vi "In.vi"   [LabVIEW 2013]
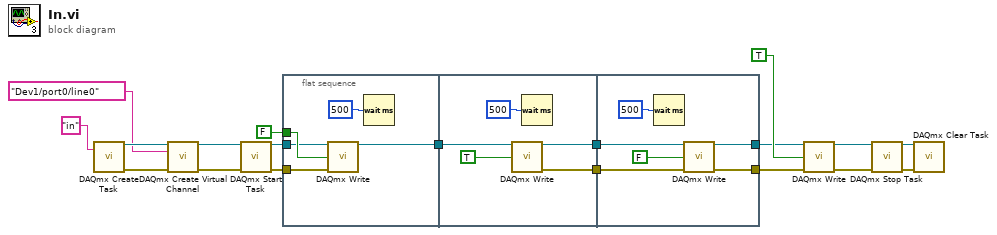
[diagram p0: block diagram]
diagram:
  n1 = call <vilib>:"DAQmx Create Task.vi"("new task name"="in") -> ("task out"=w15:refnum<k21>, "error out"=w13:errorcluster)  [unwired: 13 in]
  n2 = call-poly <vilib>:"DAQmx Create Virtual Channel.vi"("task in"=w15, "lines"=tag "Dev1/port0/line0", "error in"=w13) -> ("task out"=w12:refnum<k21>, "error out"=w11:errorcluster)  [unwired: 11 in]
  n3 = call <vilib>:"DAQmx Start Task.vi"("task/channels in"=w12, "error in"=w11) -> ("task out"=w10:refnum<k21>, "error out"=w7:errorcluster)  [unwired: 12 in]
  n4 = flat-sequence {
    tunnel: w10 -> [w20]
    tunnel: [w23] -> w19
    tunnel: w7 -> [w22]
    tunnel: FALSE ("data") -> [w21]
    tunnel: w19 -> [w28]
    tunnel: [w27] -> w18
    tunnel: [w25] -> w17
    tunnel: w18 -> [w34]
    tunnel: [w33] -> w8
    tunnel: w17 -> [w31]
    tunnel: [w30] -> w6
    frame #0 {
      n5 = call-poly <vilib>:"DAQmx Write.vi"("task/channels in"=w20, "data"=w21, "error in"=w22) -> ("task out"=w23:refnum<k21>)  [unwired: 10 in, 2 out]
      n6 = Wait (ms)(milliseconds to wait=u32 500) -> ()  [unwired: 1 out]
    }
    frame #1 {
      n7 = call-poly <vilib>:"DAQmx Write.vi"("task/channels in"=w28, "data"=TRUE) -> ("task out"=w27:refnum<k21>, "error out"=w25:errorcluster)  [unwired: 11 in, 1 out]
      n8 = Wait (ms)(milliseconds to wait=u32 500) -> ()  [unwired: 1 out]
    }
    frame #2 {
      n9 = Wait (ms)(milliseconds to wait=u32 500) -> ()  [unwired: 1 out]
      n10 = call-poly <vilib>:"DAQmx Write.vi"("task/channels in"=w34, "data"=FALSE, "error in"=w31) -> ("task out"=w33:refnum<k21>, "error out"=w30:errorcluster)  [unwired: 10 in, 1 out]
    }
  }
  n11 = call-poly <vilib>:"DAQmx Write.vi"("task/channels in"=w8, "data"=TRUE, "error in"=w6) -> ("task out"=w5:refnum<k21>, "error out"=w2:errorcluster)  [unwired: 10 in, 1 out]
  n12 = call <vilib>:"DAQmx Stop Task.vi"("task/channels in"=w5, "error in"=w2) -> ("task out"=w4:refnum<k21>, "error out"=w3:errorcluster)  [unwired: 12 in]
  n13 = call <vilib>:"DAQmx Clear Task.vi"("task in"=w4, "error in"=w3) -> ()  [unwired: 13 in, 1 out]
